vi "Dashboard Main.vi"() -> ()   [LabVIEW 2014]
uses:
  Program Files (x86)/National Instruments/LabVIEW 2014/examples/FRC/roboRIO/Vision/2015 Vision Example/Vision Support Code/Camera Types.ctl
  <vilib>/vision/Pattern Matching.llb/IMAQ Match Range Setting.ctl
  <vilib>/vision/Pattern Matching.llb/IMAQ Curve Parameters.ctl
  <vilib>/event_ctls.llb/eventvkey.ctl
  <vilib>/Rock Robotics/WPI/Dashboard/WPI_DashboardLogging Global.vi
  <vilib>/Utility/config.llb/Write Key (String).vi
  <vilib>/Utility/config.llb/Write Key (I32).vi
  <vilib>/Utility/config.llb/NI_LVConfig.lvlib
  <vilib>/vision/NI_Vision_Development_Module.lvlib
panel:
  out "Template 2":T1(plugin-control)
  in  "Camera Type":T2=enum."MS HD3000 square"
  out "ms to process":u32
  out "Particles":i32
  in  "TCP":refnum<k5>
  in  "Rec Mode":enum32{"Stop", "Record", "Playback"}(radio)
  in  "Vision":u16(ring) items=["Camera Off", "USB Camera SW", "USB Camera HW", "IP Camera"]
  out "Camera IP":string
  out "Image Message":string="Timeout in Camera Communications"
  in  "Dashboard Tab":T3(tab)
  in  "Camera Settings":T4={"Frame Rate"=30, "Compression"=30, "Size"=1} {"Frame Rate" scale=1.0..30.0; "Size" items=["640x480", "320x240", "160x120"]}
  out "MotorChart R":cluster{"Numeric":dbl, "Numeric":dbl}(graph)
  out "MotorChart L":T5(graph)
  out "MotorSliders R":cluster{"MotorSlide1":dbl, "MotorSlide2":dbl} {"MotorSlide2" scale=-1.0..1.0 scale format="%#_2e"; "MotorSlide1" scale=-1.0..1.0 scale format="%#_2e"}
  out "MotorSliders L":T6 {"MotorSlide4 2" scale=0.0..14.0 scale format="%#_2e"; "MotorSlide2" scale=-1.0..1.0 scale format="%#_2e"; "MotorSlide1" scale=-1.0..1.0 scale format="%#_2e"}
  out "Gyro":dbl(knob) scale=0.0..360.0
  out "JS1 Z":dbl(slide) scale=-1.0..1.0 scale format="%#_2e"
  out "JS1 Graph":cluster{"X":dbl, "Y":dbl}[](graph)
  out "JS1 Buttons":T7
  out "JS2 Z":dbl(slide) scale=-1.0..1.0 scale format="%#_2e"
  out "JS2 Graph":cluster{"X":dbl, "Y":dbl}[](graph)
  out "JS2 Buttons":T7
  out "Mode":T8(ring)=enum."Auto Disabled"
  in  "DB Camera Config":bool
  out "fps":dbl format="%#.1g"
  out "Mbps":dbl format="%#.1g"
  out "Mbps 2":bool
  in  "DB/String 9":string
  in  "DB/String 8":string
  in  "DB/String 7":string
  in  "DB/String 6":string
  in  "DB/String 5":string
  in  "DB/String 4":string
  in  "DB/String 3":string
  in  "DB/String 2":string
  in  "DB/String 1":string
  in  "DB/String 0":string
  in  "DB/Slider 0":dbl(slide) scale=0.0..5.0
  in  "DB/Slider 1":dbl(slide) scale=0.0..5.0
  in  "DB/Slider 2":dbl(slide) scale=0.0..5.0
  in  "DB/Slider 3":dbl(slide) scale=0.0..5.0
  out "DB/LED 3":bool
  out "DB/LED 2":bool
  out "DB/LED 1":bool
  out "DB/LED 0":bool
  in  "DB/Button 3":bool
  in  "DB/Button 2":bool
  in  "DB/Button 1":bool
  in  "DB/Button 0":bool caption="New Name"
  out "Scale":dbl
  out "Masked":T1(plugin-control)
  in  "Tote Color":T9={"Hue"={23.67058792990901, 48.923317529462665}, "Sat"={66.78571428571429, 255.0}, "Val"={48.571428571428584, 255.0}} {"Hue" scale=0.0..255.0 scale format="%#_3g"}
  out "Detected Totes":T10(array[cluster]) {"Normalized Rect"."Numeric 5" format="%#_2g"; "Normalized Rect"."Numeric 3" format="%#_2g"; "Normalized Rect"."Numeric 2" format="%#_2g"; "Normalized Rect"."Numeric" format="%#_2g"}
  out "Sorted Scores":T11(array[cluster]) {"Correlation" format="%#_3g"; "Scale %" format="%#_3g"; "Score" format="%#_3g"}
  in  "Annotate":bool=TRUE
  in  "Score Threshold":dbl=75.0
  out "RightSide":dbl
  out "LeftSide":dbl
  in  "Test Slider":dbl(slide) scale=0.0..100.0 scale format="%#_3g"
  in  "On/Off":bool caption="Solenoid"
  in  "Test Name":u16(ring) items=["Select the test to run...", "Example Test", "-------------------------------", "List of tests is built in robot code.", "Replace with your own automated tests."]
  in  "Test Tree":string(tree)
  in  "Motor":cluster{"Value":dbl, "Enable":bool} {"Value" scale=-1.0..1.0 scale format="%#_3g"}
  out "Progress":T12 {"Test Progress" scale=0.0..100.0}
  in  "Rev/Fwd":cluster{"Forward":bool, "Reverse":bool}
  in  "Test Ring":u16(ring) items=["Monochrome", "Color"]
  in  "Listbox":i32(listbox)
  out "Tree":string(tree)
  out "Camera Image":T1(plugin-control)
  out "Boolean":bool
  # "Left"
  # "Front"
  # "Right"
  # "Battery"
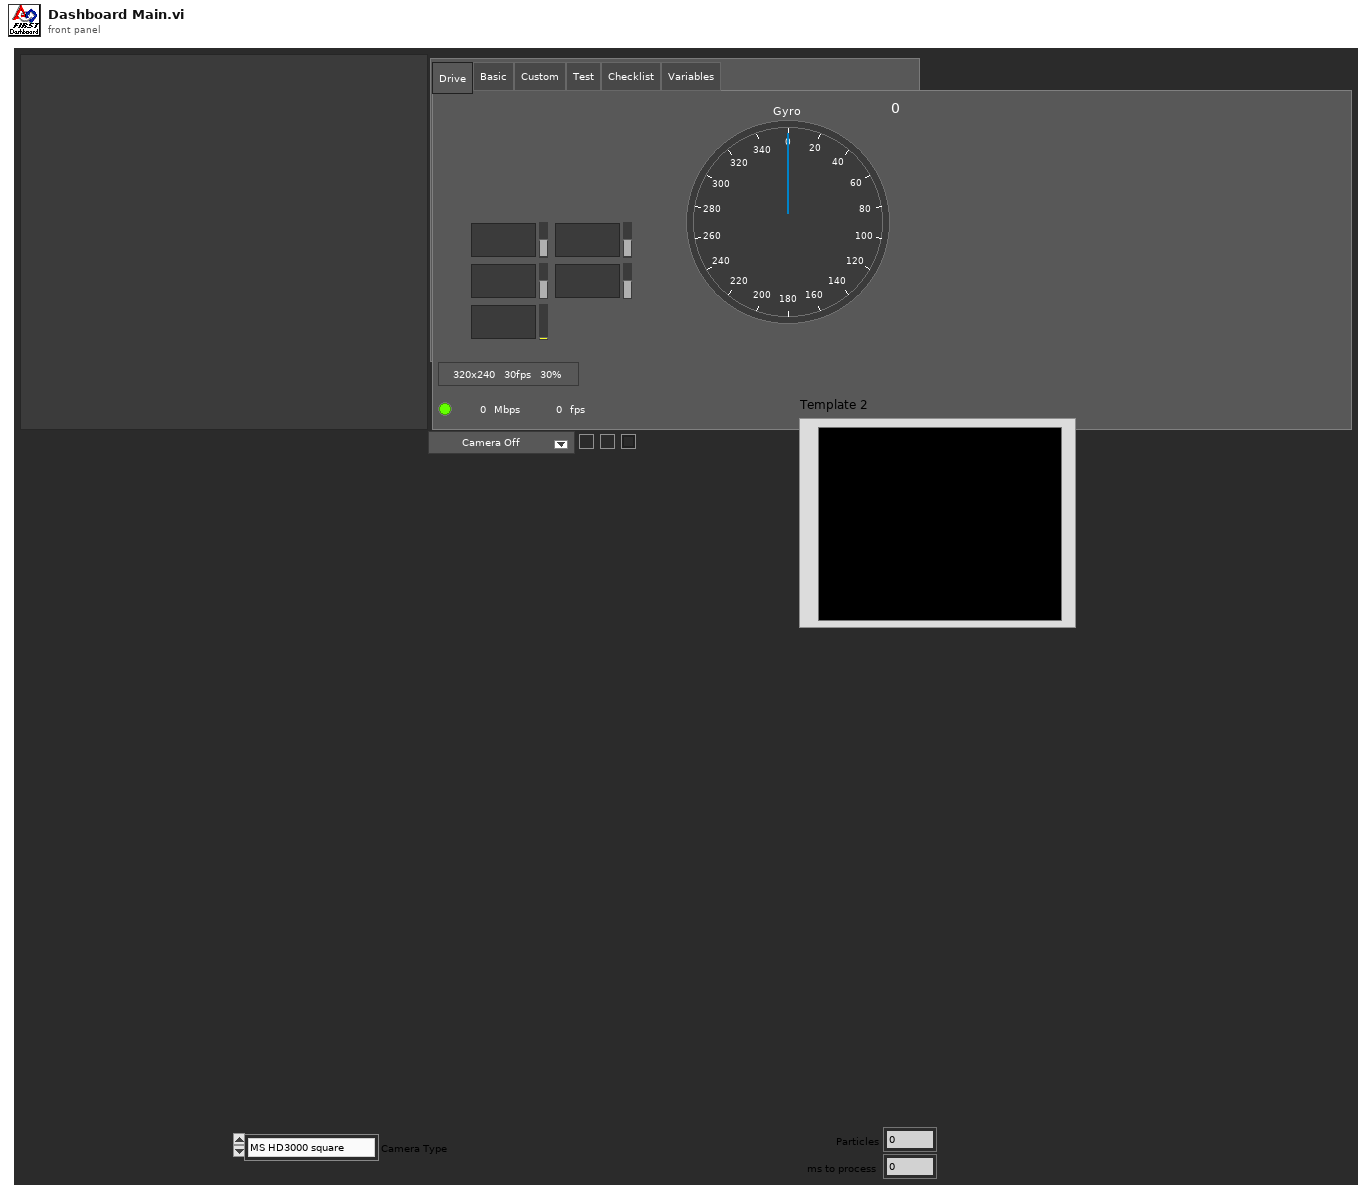
[diagram p1: front panel]
types:
  T1 = typedef "IMAQ Image.ctl" = refnum<image>
  T2 = typedef "Camera Types.ctl" = enum16{"206", "1011", "1013", "MS HD3000 square", "MS HD3000 640x480"}
  T3 = enum32{"Drive", "Basic", "Custom", "Test", "Checklist", "Variables"}
  T4 = cluster{"Frame Rate":i32, "Compression":i32, "Size":u16}
  T5 = cluster{"Numeric":dbl, "Numeric":dbl, "Battery V":dbl}
  T6 = cluster{"MotorSlide1":dbl, "MotorSlide2":dbl, "MotorSlide4 2":dbl}
  T7 = cluster{bool, bool, bool, bool, bool, bool, bool, bool, bool, bool, bool, bool}
  T8 = enum8{"Tele-Op Disabled", "Tele-Op Enabled", "Auto Disabled", "Auto Enabled", "Test Disabled", "Test Enabled", "Disconnected", "No Code", "E-Stop"}
  T9 = cluster{"Hue":cluster{dbl, dbl}, "Sat":cluster{dbl, dbl}, "Val":cluster{dbl, dbl}}
  T10 = cluster{"Distance (ft)":dbl, "Center":cluster{dbl, dbl}, "Normalized Rect":cluster{"Numeric":dbl, "Numeric 2":dbl, "Numeric 3":dbl, "Numeric 5":dbl}}[]
  T11 = cluster{"Rectangle":cluster{"Numeric":dbl, "Numeric 2":dbl, "Numeric 3":dbl, "Numeric 5":dbl}, "Scale %":dbl, "Score":dbl, "Correlation":dbl}[]
  T12 = cluster{"Test Progress":u8, "Test Progress Text":string}
  T13 = cluster{"Rotation":bool, "Scale":bool, "Occlusion":bool, "Reserved":bool, "Reserved":bool, "Reserved":bool}
  T14 = typedef "IMAQ Curve Parameters.ctl" = cluster{"Extraction Mode":u32, "Edge Threshold":i32, "Edge Filter Size":u32, "Min Length":i32, "Row Search Step Size":i32, "Col Search Step Size":i32, "Max Endpoint Gap":i32, "Closed":bool, "Subpixel":bool}
  T15 = typedef "IMAQ Match Range Setting.ctl" = cluster{"Match Constraints":u32, "Min":dbl, "Max":dbl}
  T16 = typedef "Image Type" = u32
  T17 = typedef "Particle Parameters" = i32
  T18 = cluster{"Error Strings":string, "Disable Counts":cluster{u16, u16}, "Rail Faults":cluster{u16, u16, u16}, "Robot IP":string, "DB Mode":u8, "Event Info":cluster{"Name":string, "Type":u8, "Number":u16, "Replay":u8}, "Camera Addr":string}
  T19 = cluster{"Storage":cluster{"Disk Free":u64, "RAM Block":u32, "RAM free":u32}, "CPU Utilization":cluster{"CPU % ISR":sgl, "CPU % Time Crit":sgl, "CPU % Timed Str":sgl, "CPU % High":sgl, "CPU % Above":sgl, "CPU % Normal":sgl, "CPU % Low":sgl}, "CAN":cluster{"% Bus Utilization":sgl, "Bus Off Cnt":u32, "TX_FIFO Full Cnt":u32, "Receive Error Cnt":u8, "Transmit Error Cnt":u8}, "HID":cluster{"HID Outputs":u32, "Rumble Low":u16, "Rumble High":u16}[]}
  T20 = cluster{"Status bits":cluster{"Test Mode":bool, "Autonomous":bool, "Enabled":bool, "Code Start":bool, "Brownout":bool, "Reserved 2":bool, "Reserved 3":bool, "E-Stop":bool}, "Code Trace":cluster{"Disabled":bool, "TeleOp":bool, "Auto":bool, "Test":bool}, "Controller Type":enum16{"unknown", "cRIO", "roboRio"}, "Code?":enum16{"unknown", "noCode", "code"}, "Battery V":dbl}
  T21 = cluster{"Control Bits":cluster{"TestMode":bool, "Autonomous":bool, "Enabled":bool, "FMS Present":bool, bool, bool, bool, "E-Stop":bool}, "Team Station ":u8, "Countdown":sgl, "Joystick Values":cluster{"Axes":dbl[], "Buttons":bool[], "POVs":i16[]}[]}
  T22 = cluster{"Axes":dbl[], "Buttons":bool[], "POVs":i16[]}[]
  T23 = cluster{"Axes":dbl[], "Buttons":bool[], "POVs":i16[]}
  T24 = cluster{"Buttons[0]":bool, "Buttons[1]":bool, "Buttons[2]":bool, "Buttons[3]":bool, "Buttons[4]":bool, "Buttons[5]":bool, "Buttons[6]":bool, "Buttons[7]":bool, "Buttons[8]":bool, "Buttons[9]":bool, "Buttons[10]":bool, "Buttons[11]":bool}
  T25 = cluster{"[0]":dbl, "[1]":dbl, "[2]":dbl, "[3]":dbl}
  T26 = cluster{"[0]":dbl, "[1]":dbl, "[2]":dbl, "[3]":dbl, "[4]":dbl}
  T27 = typedef "ROI Descriptor" = cluster{"Global Rectangle":i32[], "Contours":cluster{"ID":enum32{"External", "Internal"}, "Type":u32, "Coordinates":i32[]}[]}
  T28 = typedef "IMAQ GM Match Report.ctl" = cluster{"Position":cluster{"x":sgl, "y":sgl}, "Angle":sgl, "Scale":sgl, "Score":sgl, "Bounding Box":cluster{"x":sgl, "y":sgl}[], "Contrast Reversed":bool, "Occlusion %":sgl, "Template Target Curve Score":sgl, "Target Template Curve Score":sgl, "Correlation Score":sgl}
  T29 = cluster{cluster{"[0]":dbl, "[1]":dbl, "[2]":dbl, "[3]":dbl}, "Position":cluster{"x":sgl, "y":sgl}, "Bounding Box":cluster{"x":sgl, "y":sgl}[], "Scale":sgl, "Score":sgl, "Correlation Score":sgl}
  T30 = cluster{"Rectangle":cluster{"Numeric":dbl, "Numeric 2":dbl, "Numeric 3":dbl, "Numeric 5":dbl}, "Scale":dbl, "Score":dbl, "Correlation":dbl}[]
  T31 = cluster{"Found Totes[0]":cluster{"Distance (ft)":dbl, "Center":cluster{dbl, dbl}, "Normalized Rect":cluster{"Numeric":dbl, "Numeric 2":dbl, "Numeric 3":dbl, "Numeric 5":dbl}}, "Found Totes[1]":cluster{"Distance (ft)":dbl, "Center":cluster{dbl, dbl}, "Normalized Rect":cluster{"Numeric":dbl, "Numeric 2":dbl, "Numeric 3":dbl, "Numeric 5":dbl}}, "Found Totes[2]":cluster{"Distance (ft)":dbl, "Center":cluster{dbl, dbl}, "Normalized Rect":cluster{"Numeric":dbl, "Numeric 2":dbl, "Numeric 3":dbl, "Numeric 5":dbl}}, "Found Totes[3]":cluster{"Distance (ft)":dbl, "Center":cluster{dbl, dbl}, "Normalized Rect":cluster{"Numeric":dbl, "Numeric 2":dbl, "Numeric 3":dbl, "Numeric 5":dbl}}, "Found Totes[4]":cluster{"Distance (ft)":dbl, "Center":cluster{dbl, dbl}, "Normalized Rect":cluster{"Numeric":dbl, "Numeric 2":dbl, "Numeric 3":dbl, "Numeric 5":dbl}}, "Found Totes[5]":cluster{"Distance (ft)":dbl, "Center":cluster{dbl, dbl}, "Normalized Rect":cluster{"Numeric":dbl, "Numeric 2":dbl, "Numeric 3":dbl, "Numeric 5":dbl}}, "Found Totes[6]":cluster{"Distance (ft)":dbl, "Center":cluster{dbl, dbl}, "Normalized Rect":cluster{"Numeric":dbl, "Numeric 2":dbl, "Numeric 3":dbl, "Numeric 5":dbl}}, "Found Totes[7]":cluster{"Distance (ft)":dbl, "Center":cluster{dbl, dbl}, "Normalized Rect":cluster{"Numeric":dbl, "Numeric 2":dbl, "Numeric 3":dbl, "Numeric 5":dbl}}, "Found Totes[8]":cluster{"Distance (ft)":dbl, "Center":cluster{dbl, dbl}, "Normalized Rect":cluster{"Numeric":dbl, "Numeric 2":dbl, "Numeric 3":dbl, "Numeric 5":dbl}}}
  T32 = cluster{"Distance (ft)":dbl, "Center":cluster{dbl, dbl}, "Normalized Rect":cluster{"Numeric":dbl, "Numeric 2":dbl, "Numeric 3":dbl, "Numeric 5":dbl}}
  T33 = cluster{"Sorted Scores[0]":cluster{"Rectangle":cluster{"Numeric":dbl, "Numeric 2":dbl, "Numeric 3":dbl, "Numeric 5":dbl}, "Scale":dbl, "Score":dbl, "Correlation":dbl}, "Sorted Scores[1]":cluster{"Rectangle":cluster{"Numeric":dbl, "Numeric 2":dbl, "Numeric 3":dbl, "Numeric 5":dbl}, "Scale":dbl, "Score":dbl, "Correlation":dbl}, "Sorted Scores[2]":cluster{"Rectangle":cluster{"Numeric":dbl, "Numeric 2":dbl, "Numeric 3":dbl, "Numeric 5":dbl}, "Scale":dbl, "Score":dbl, "Correlation":dbl}, "Sorted Scores[3]":cluster{"Rectangle":cluster{"Numeric":dbl, "Numeric 2":dbl, "Numeric 3":dbl, "Numeric 5":dbl}, "Scale":dbl, "Score":dbl, "Correlation":dbl}, "Sorted Scores[4]":cluster{"Rectangle":cluster{"Numeric":dbl, "Numeric 2":dbl, "Numeric 3":dbl, "Numeric 5":dbl}, "Scale":dbl, "Score":dbl, "Correlation":dbl}, "Sorted Scores[5]":cluster{"Rectangle":cluster{"Numeric":dbl, "Numeric 2":dbl, "Numeric 3":dbl, "Numeric 5":dbl}, "Scale":dbl, "Score":dbl, "Correlation":dbl}, "Sorted Scores[6]":cluster{"Rectangle":cluster{"Numeric":dbl, "Numeric 2":dbl, "Numeric 3":dbl, "Numeric 5":dbl}, "Scale":dbl, "Score":dbl, "Correlation":dbl}, "Sorted Scores[7]":cluster{"Rectangle":cluster{"Numeric":dbl, "Numeric 2":dbl, "Numeric 3":dbl, "Numeric 5":dbl}, "Scale":dbl, "Score":dbl, "Correlation":dbl}, "Sorted Scores[8]":cluster{"Rectangle":cluster{"Numeric":dbl, "Numeric 2":dbl, "Numeric 3":dbl, "Numeric 5":dbl}, "Scale":dbl, "Score":dbl, "Correlation":dbl}}
  T34 = cluster{"Rectangle":cluster{"Numeric":dbl, "Numeric 2":dbl, "Numeric 3":dbl, "Numeric 5":dbl}, "Scale":dbl, "Score":dbl, "Correlation":dbl}
  T35 = cluster{"Numeric":dbl, "Numeric 2":dbl, "Numeric 3":dbl, "Numeric 5":dbl}
  T36 = typedef "NI_LVConfig.lvlib/Config Data RefNum.ctl" = refnum<k1>
  T37 = cluster{"Operation":enum16{"Update", "Clear"}, "Color Box":u32}[]
  T38 = typedef "eventvkey.ctl" = enum16{"ASCII", "Enter", "Return", "Shift", "Ctrl", "Alt", "Cmd", "Opt", "Caps", "NumLock", "Clear", "Break", "Up", "Down", "Left", "Right", "Insert", "Delete", "Home", "End", "PageUp", "PageDown", "Escape", "Help", "Pause", "ScrollLock", "F1", "F2", "F3", "F4", "F5", "F6", "F7", "F8", "F9", "F10", "F11", "F12", "F13", "F14", "F15", "F16", "F17", "F18", "F19", "F20", "F21", "F22", "F23", "F24", "Play", "VolumeUp", "VolumeDown", "Mute", "Two Byte Char"}
  T39 = cluster{"Image Size":bool, "Image Type":bool, "Pixel Value":bool, "ROI Information":bool, "Zoom Factor":bool}
  T40 = enum8{"Enabled", "Disabled", "Disabled and Grayed Out"}
  T41 = cluster{"Operation":enum16{"Update", "Clear"}, "Color Box":u32}
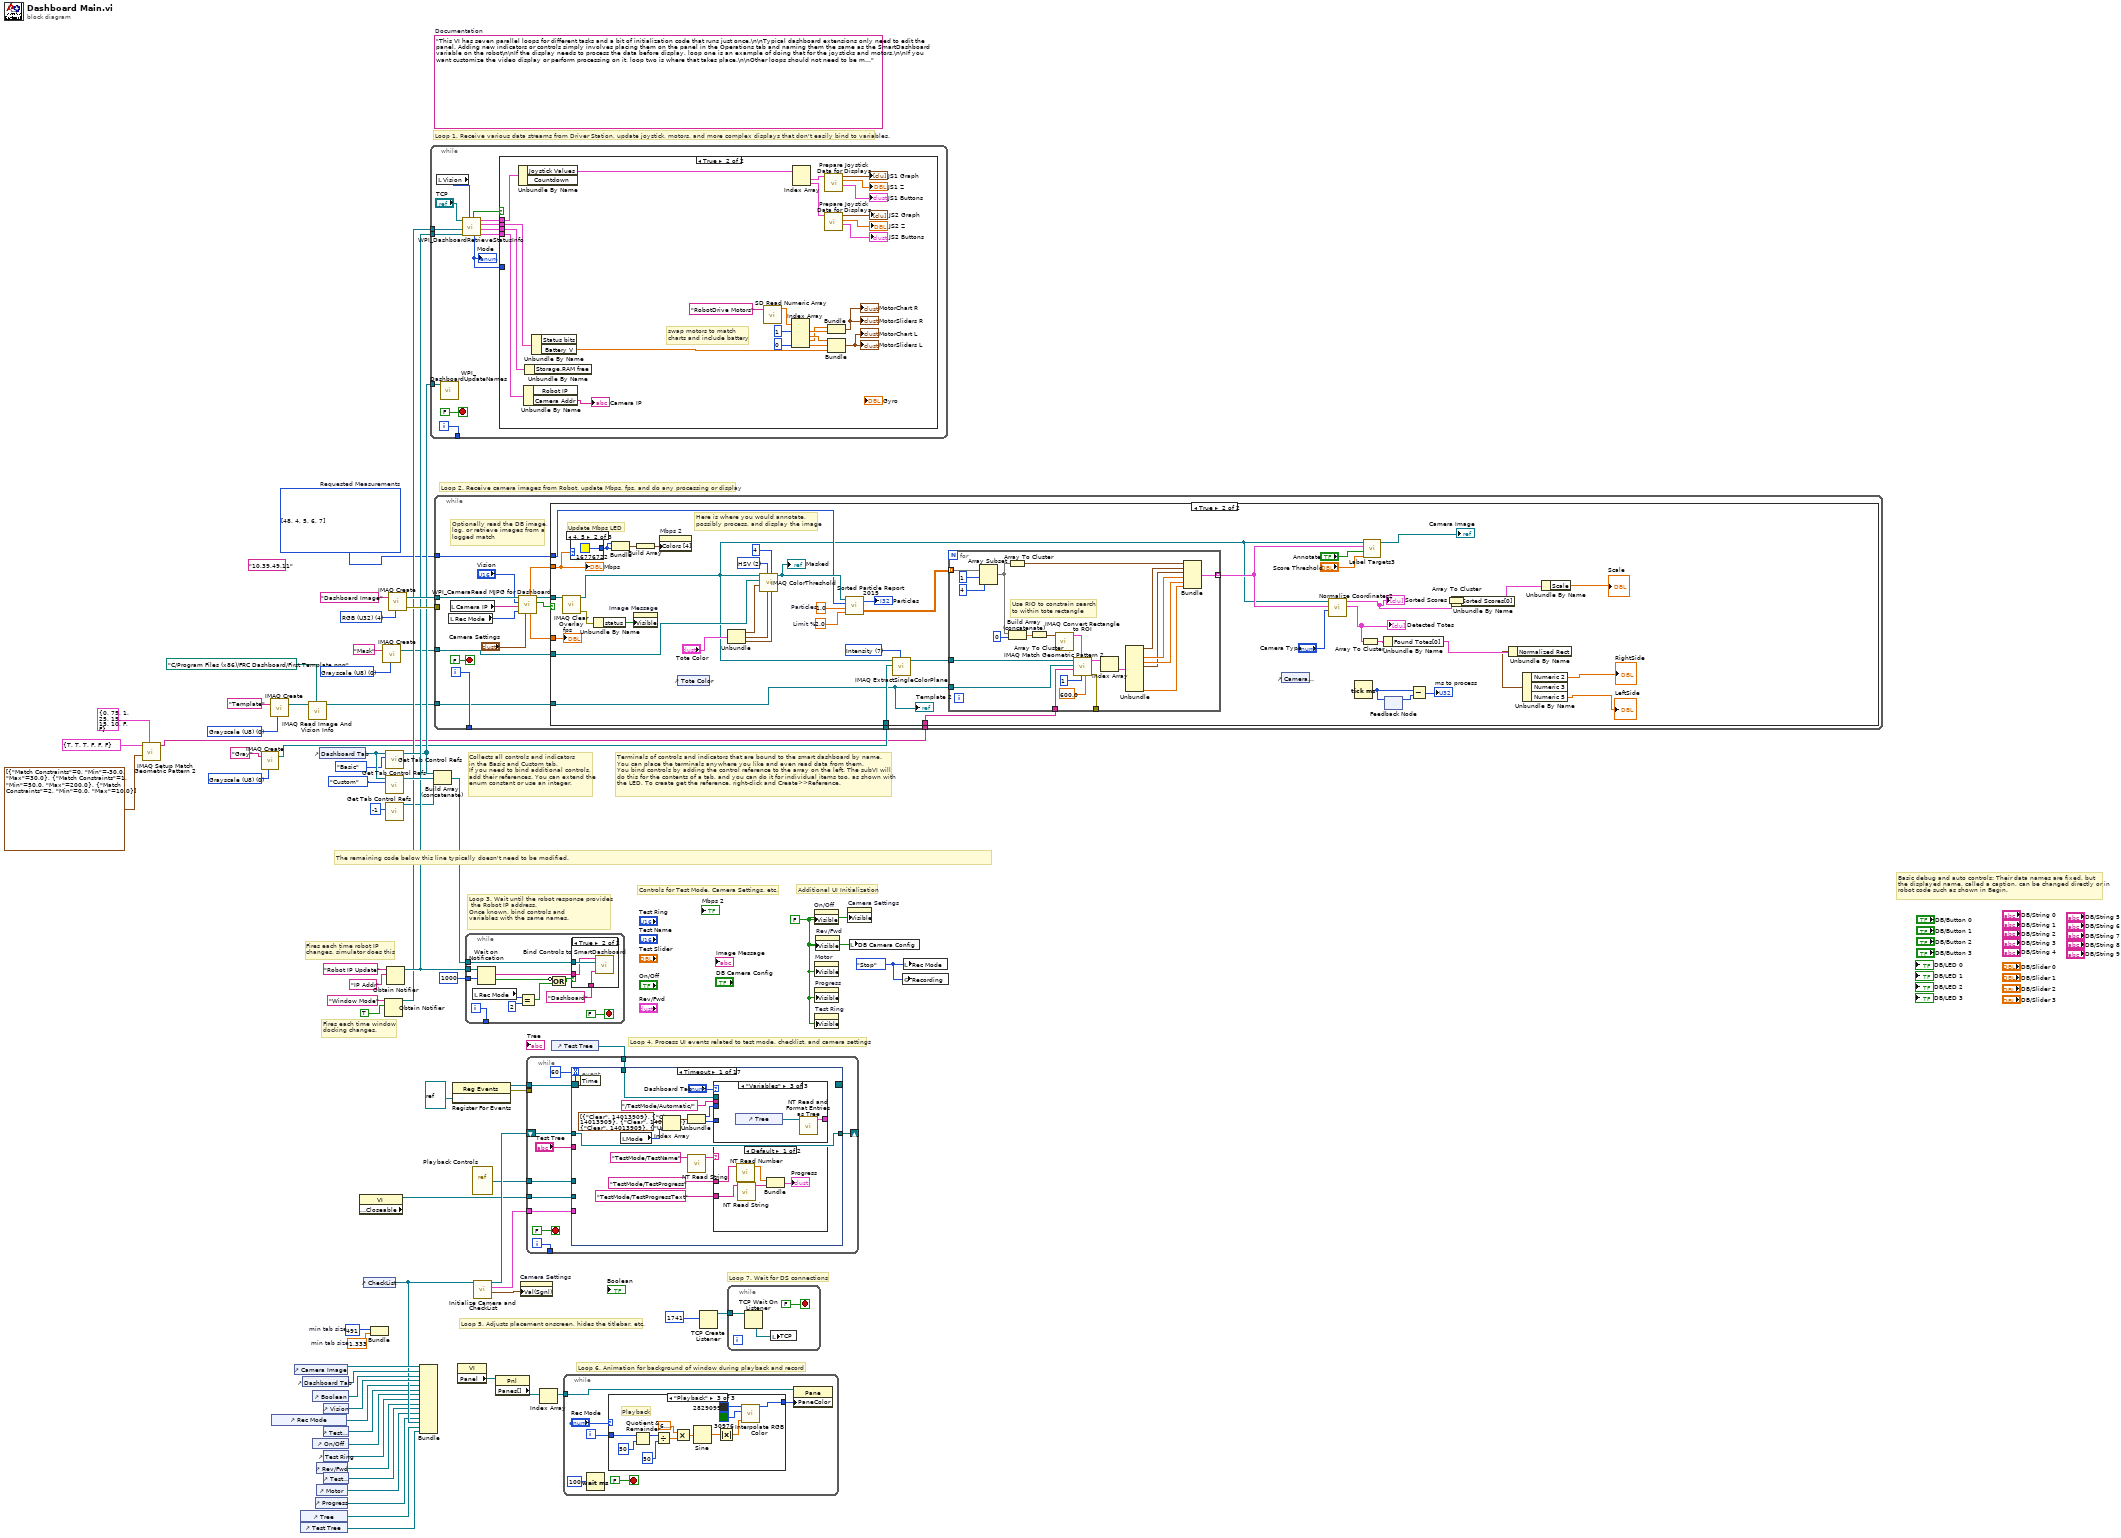
[diagram p0: block diagram]
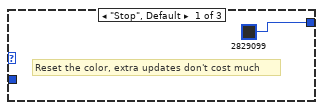
[diagram p3: hidden frame]
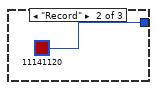
[diagram p4: hidden frame]
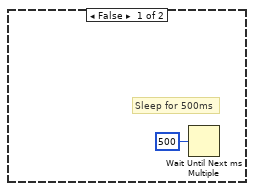
[diagram p6: hidden frame]
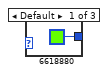
[diagram p7: hidden frame]
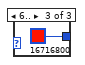
[diagram p8: hidden frame]
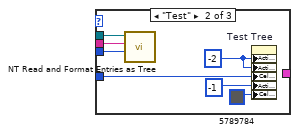
[diagram p10: hidden frame]
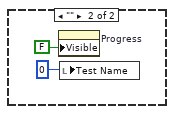
[diagram p11: hidden frame]
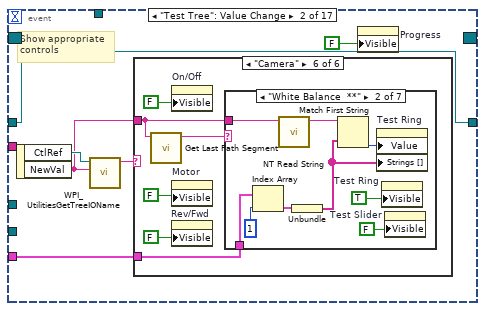
[diagram p12: hidden frame]
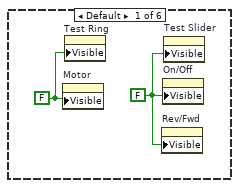
[diagram p13: hidden frame]
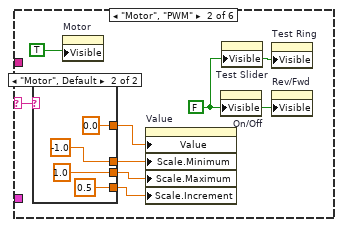
[diagram p14: hidden frame]
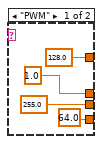
[diagram p15: hidden frame]
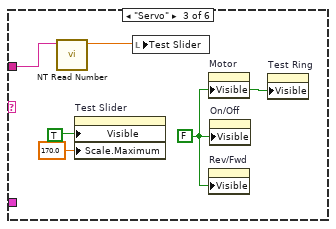
[diagram p16: hidden frame]
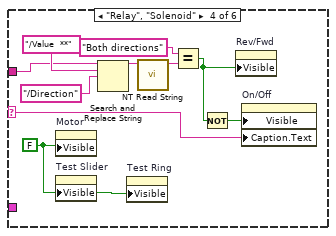
[diagram p17: hidden frame]
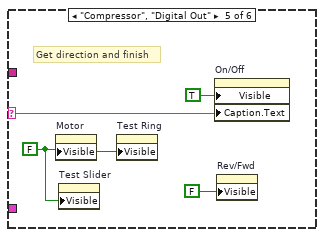
[diagram p18: hidden frame]
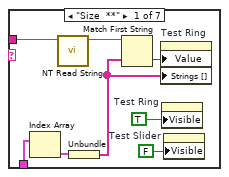
[diagram p19: hidden frame]
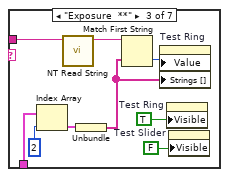
[diagram p20: hidden frame]
diagram:
  (unwired) "10.39.49.11" ("Camera IP")
  w10 = T16 0 items=["Grayscale (U8)", "Grayscale (I16)", "Grayscale (SGL)", "Complex (CSG)", "RGB (U32)", "HSL (U32)", "RGB (U64)", "Grayscale (U16)"] ("Image Type")
  w14 = T16 0 items=["Grayscale (U8)", "Grayscale (I16)", "Grayscale (SGL)", "Complex (CSG)", "RGB (U32)", "HSL (U32)", "RGB (U64)", "Grayscale (U16)"] ("Image Type")
  w15 = T17[] [48, 4, 5, 6, 7] items=["Center of Mass X", "Center of Mass Y", "First Pixel X", "First Pixel Y", "Bounding Rect Left", "Bounding Rect Top", "Bounding Rect Right", "Bounding Rect Bottom", "Max Feret Diameter Start X", "Max Feret Diameter Start Y", "Max Feret Diameter End X", "Max Feret Diameter End Y", "Max Horiz. Segment Length Left", "Max Horiz. Segment Length Right", "Max Horiz. Segment Length Row", "-", "Bounding Rect Width", "Bounding Rect Height", "Bounding Rect Diagonal", "Perimeter", "Convex Hull Perimeter", "Holes' Perimeter", "Max Feret Diameter", "Equivalent Ellipse Major Axis", "Equivalent Ellipse Minor Axis", "Equivalent Ellipse Minor Axis (Feret)", "Equivalent Rect Long Side", "Equivalent Rect Short Side", "Equivalent Rect Diagonal", "Equivalent Rect Short Side (Feret)", "Average Horiz. Segment Length", "Average Vert. Segment Length", "Hydraulic Radius", "Waddel Disk Diameter", "-", "Area", "Holes' Area", "Particle & Holes' Area", "Convex Hull Area", "Image Area", "-", "Number of Holes", "Number of Horiz. Segments", "Number of Vert. Segments", "-", "Orientation", "Max Feret Diameter Orientation", "-", "% Area/Image Area", "% Area/(Particle & Holes' Area)", "Ratio of Equivalent Ellipse Axes", "Ratio of Equivalent Rect Sides", "-", "Elongation Factor", "Compactness Factor", "Heywood Circularity Factor", "Type Factor", "-", "Sum X", "Sum Y", "Sum XX", "Sum XY", "Sum YY", "Sum XXX", "Sum XXY", "Sum XYY", "Sum YYY", "-", "Moment of Inertia XX", "Moment of Inertia XY", "Moment of Inertia YY", "Moment of Inertia XXX", "Moment of Inertia XXY", "Moment of Inertia XYY", "Moment of Inertia YYY", "Norm. Moment of Inertia XX", "Norm. Moment of Inertia XY", "Norm. Moment of Inertia YY", "Norm. Moment of Inertia XXX", "Norm. Moment of Inertia XXY", "Norm. Moment of Inertia XYY", "Norm. Moment of Inertia YYY", "Hu Moment 1", "Hu Moment 2", "Hu Moment 3", "Hu Moment 4", "Hu Moment 5", "Hu Moment 6", "Hu Moment 7"]  # Requested Measurements
  w18 = T16 0 items=["Grayscale (U8)", "Grayscale (I16)", "Grayscale (SGL)", "Complex (CSG)", "RGB (U32)", "HSL (U32)", "RGB (U64)", "Grayscale (U16)"] ("Image Type")
  w40 = 491  # min tab size
  w39 = 1.333  # min tab size
  w48 = enum32{"Stop", "Record", "Playback"}."Stop" ("Rec Mode")
  w24 = FALSE ("Visible")
  (unwired) "This VI has seven parallel loops for different tasks and a bit of initialization code that runs just once.\n\nTypical dashboard extensions only need to edit the panel. Adding new indicators or controls simply involves placing them on the panel in the Operations tab and naming them the same as the SmartDashboard variable on the robot\n\nIf the display needs to process the data before display, loop one is an example of doing that for the joysticks and motors.\n\nIf you want customize the video display or perform processing on it, loop two is where that takes place.\n\nOther loops should not need to be modified. They are pretty standard, and document the task they perform."  # Documentation
  w68 = T16 4 items=["Grayscale (U8)", "Grayscale (I16)", "Grayscale (SGL)", "Complex (CSG)", "RGB (U32)", "HSL (U32)", "RGB (U64)"] ("Image Type")
  # "Loop 7. Wait for DS connections"
  # "Basic debug and auto controls: Their data names are fixed, but\nthe displayed name, called a caption, can be changed directly or in\nrobot code such as shown in Begin."
  # "Controls for Test Mode, Camera Settings, etc."
  # "Additional UI Initialization"
  # "Loop 6. Animation for background of window during playback and record"
  # "Fires each time robot IP\nchanges, simulator does this"
  # "Fires each time window\ndocking changes."
  # "Collects all controls and indicators\nin the Basic and Custom tab.\nIf you need to bind additional controls,\nadd their references. You can extend the\nenum constant or use an integer."
  # "The remaining code below this line typically doesn't need to be modified."
  # "Loop 4. Process UI events related to test mode, checklist, and camera settings"
  # "Terminals of controls and indicators that are bound to the smart dashboard by name.\nYou can place the terminals anywhere you like and even read data from them.\nYou bind controls by adding the control reference to the array on the left. The subVI will\ndo this for the contents of a tab, and you can do it for individual items too, as shown with\nthe LED. To create get the reference, right-click and Create>>Reference."
  # "Loop 3. Wait until the robot response provides\n the Robot IP address.\nOnce known, bind controls and\nvariables with the same names."
  # "Loop 5. Adjusts placement onscreen, hides the titlebar, etc."
  # "Loop 1. Receive various data streams from Driver Station, update joystick, motors, and more complex displays that don't easily bind to variables."
  # "Loop 2. Receive camera images from Robot, update Mbps, fps, and do any processing or display"
  n1 = call "IMAQ Setup Match Geometric Pattern 2"("Curve Parameters"=T14 {"Extraction Mode"=0, "Edge Threshold"=75, "Edge Filter Size"=1, "Min Length"=25, "Row Search Step Size"=15, "Col Search Step Size"=15, "Max Endpoint Gap"=10, "Closed"=FALSE, "Subpixel"=FALSE}, "Range Settings"=T15[] [{"Match Constraints"=0, "Min"=-30.0, "Max"=30.0}, {"Match Constraints"=1, "Min"=50.0, "Max"=200.0}, {"Match Constraints"=2, "Min"=0.0, "Max"=10.0}], "Match Mode"=T13 {"Rotation"=TRUE, "Scale"=TRUE, "Occlusion"=TRUE, "Reserved"=FALSE, "Reserved"=FALSE, "Reserved"=FALSE}) -> ("Match Geometric Pattern 2 Setup Data"=w4:string)  [unwired: 7 in, 1 out]
  n2 = call "IMAQ Create"("Image Name"="Gray", "Image Type"=w10) -> ("New Image"=w8:T1)  [unwired: 2 in, 2 out]
  n3 = call "IMAQ Create"("Image Name"="Template", "Image Type"=w14) -> ("New Image"=w12:T1)  [unwired: 2 in, 2 out]
  n4 = control-ref of="Rec Mode"() -> (w30:refnum<vi>)
  n5 = control-ref of="Camera Image"() -> (w43:refnum<vi>)
  n6 = control-ref of="Tree"() -> (w34:refnum<vi>)
  n7 = control-ref of="Test Tree"() -> (w33:refnum<vi>)
  n8 = control-ref of="Dashboard Tab"() -> (w42:refnum<vi>)
  n9 = call "IMAQ Read Image And Vision Info"("File Path"=path "C:/Program Files (x86)/FRC Dashboard/First Template.png", "Image"=w12) -> ("Image Out"=w11:T1)  [unwired: 2 in, 7 out]
  n10 = control-ref of="Boolean"() -> (w38:refnum<vi>)
  n11 = control-ref of="On/Off"() -> (w28:refnum<vi>)
  n12 = control-ref of="Progress"() -> (w25:refnum<vi>)
  n13 = control-ref of="Rev/Fwd"() -> (w26:refnum<vi>)
  n14 = control-ref of="Motor"() -> (w31:refnum<vi>)
  n15 = control-ref of="Dashboard Tab"() -> (w46:refnum<vi>)
  n16 = control-ref of="Test Slider"() -> (w29:refnum<vi>)
  n17 = control-ref of="Vision"() -> (w41:refnum<vi>)
  n18 = control-ref of="Test Ring"() -> (w27:refnum<vi>)
  n19 = control-ref of="Test Name"() -> (w32:refnum<vi>)
  n20 = property class="VI" props=["Front Panel.Closeable"]() -> (reference out=w47:refnum<vi>)  [unwired: 2 in, 2 out]
  n21 = control-ref of="CheckList"() -> (w35:refnum<vi>)
  n22 = Bundle("min tab size"=w40, "min tab size"=w39) -> ()  [unwired: 1 in, 1 out]
  n23 = call "IMAQ Create"("Image Name"="Mask", "Image Type"=w18) -> ("New Image"=w16:T1)  [unwired: 2 in, 2 out]
  n24 = Obtain Notifier(name (unnamed)="Window Mode", notification data type=TRUE) -> (notifier out=w21:refnum<notifier>)  [unwired: 2 in, 2 out]
  n25 = call <vilib>:"Get Tab Control Refs.vi"("Page Index"=T3."Basic" ("Dashboard Tab"), "TabControl in"=w46) -> ("ControlsOnPage"=w22:refnum<vi>[])  [unwired: 9 in]
  n26 = call <vilib>:"Get Tab Control Refs.vi"("Page Index"=T3."Custom" ("Dashboard Tab"), "TabControl in"=w46) -> ("ControlsOnPage"=w45:refnum<vi>[])  [unwired: 9 in]
  n27 = call <vilib>:"Get Tab Control Refs.vi"("Page Index"=-1) -> ("ControlsOnPage"=w2:refnum<vi>[])  [unwired: 10 in]
  n28 = Obtain Notifier(name (unnamed)="Robot IP Update", notification data type="IP Addr" ("name (unnamed)")) -> (notifier out=w23:refnum<notifier>)  [unwired: 2 in, 2 out]
  n29 = call "IMAQ Create"("Image Name"="Dashboard Image", "Image Type"=w68) -> ("New Image"=w66:T1, "error out"=w65:errorcluster)  [unwired: 2 in, 1 out]
  n30 = Bundle("Camera Image"=w43, "Dashboard Tab"=w42, "Boolean"=w38, "Vision"=w41, "Rec Mode"=w30, "Test Slider"=w29, "On/Off"=w28, "Test Ring"=w27, "Rev/Fwd"=w26, "Test Name"=w32, "Motor"=w31, "Progress"=w25, "CheckList"=w35, "Tree"=w34, "Test Tree"=w33) -> ()  [unwired: 1 in, 1 out]
  n31 = while {
    tunnel: [w80] -> _
    tunnel: w23 -> [w74]
    tunnel: w22 -> [w73]
    tunnel: w21 -> [w69]
    i -> [w80]
    stop <- FALSE stop-if-true
    n32 = local read "Vision"() -> (w71:u16)
    n33 = call <vilib>:"WPI_DashboardUpdateNames.vi"("Controls on Tab"=w73) -> ()  [unwired: 11 in]
    n34 = call <vilib>:"WPI_DashboardRetrieveStatusInfo.vi"("Vision"=w71, "Binding Refnum"=w74, "Window Mode Notifier"=w69, "TCP Cnx"="TCP") -> ("Power and Errors"=w75:T18, "Robot Metrics"=w78:T19, "Status Info"=w79:T20, "Control Info"=w76:T21, "Robot Mode"=w72:T8, "Process?"=w77:bool)  [unwired: 2 in]
    "Mode" <- w72
    n35 = case shown="True" w77 {
      tunnel: w79 -> [_ w106]
      tunnel: w78 -> [_ w105]
      tunnel: w76 -> [_ w104]
      tunnel: w75 -> [_ w103]
      tunnel: w72 -> [_ _]
      frame False {
      }
      frame True {
        # "swap motors to match\ncharts and include battery"
        n36 = Unbundle By Name(w104) -> ("Joystick Values"=w91:T22)  [unwired: 1 out]
        n37 = Unbundle By Name(w103) -> ("Camera Addr"=→"Camera IP":string)  [unwired: 1 out]
        n38 = Unbundle By Name(w105) -> ()  [unwired: 1 out]
        n39 = Unbundle By Name(w106) -> ("Battery V"=w92:dbl)  [unwired: 1 out]
        n40 = call <vilib>:"SD Read Numeric Array.vi"("Name"="RobotDrive Motors") -> ("Numeric Array"=w94:dbl[])  [unwired: 8 in, 2 out]
        n41 = Index Array(array=w94, index #1=1, index #4=0) -> (element #1=w98:dbl, element #2=w99:dbl, element #3=w97:dbl, element #4=w102:dbl)  [unwired: 2 in]
        n42 = Index Array(array=w91) -> (element #1=w90:T23, element #2=w85:T23)  [unwired: 2 in]
        n43 = call "Prepare Joystick Data for Displays.vi"("Joystick Values"=w85) -> ("Buttons"=→"JS2 Buttons":T24, "Z Axis"=→"JS2 Z":dbl, "Cartesian Data"=→"JS2 Graph":cluster{"X axis":dbl, "X axis":dbl}[])  [unwired: 8 in]
        n44 = call "Prepare Joystick Data for Displays.vi"("Joystick Values"=w90) -> ("Buttons"=→"JS1 Buttons":T24, "Z Axis"=→"JS1 Z":dbl, "Cartesian Data"=→"JS1 Graph":cluster{"X axis":dbl, "X axis":dbl}[])  [unwired: 8 in]
        n45 = Bundle("Numeric"=w97, "Numeric"=w98) -> (→"MotorChart R" →"MotorSliders R":cluster{"Numeric":dbl, "Numeric":dbl})  [unwired: 1 in]
        n46 = Bundle("Numeric"=w99, "Numeric"=w102, "Battery V"=w92) -> (→"MotorChart L" →"MotorSliders L":T5)  [unwired: 1 in]
      }
    }
  }
  n47 = Build Array (concatenate)(w22, w45, w2) -> (w44:refnum<vi>[])
  n48 = while {
    tunnel: w66 -> [w120]
    tunnel: w65 -> [_]
    tunnel: [w121] -> _
    tunnel: w16 -> [w112]
    tunnel: w15 -> [w111]
    tunnel: w11 -> [w110]
    tunnel: w8 -> [w109]
    tunnel: w4 -> [w108]
    i -> [w121]
    stop <- FALSE stop-if-true
    # "Optionally read the DB image,\nlog, or retrieve images from a\nlogged match"
    n49 = local read "Rec Mode"() -> (w114:enum32{"Stop", "Record", "Playback"})
    n50 = local read "Camera IP"() -> (w107:string)
    n51 = call <vilib>:"WPI_CameraRead MJPG for Dashboard.vi"("Camera Settings"="Camera Settings", "Rec Mode"=w114, "Camera IP"=w107, "Camera Mode"="Vision", "Refnum in"=w120) -> ("Active"=w118:bool, "Refnum out"=w119:T1, "FPS"=w117:dbl, "Bandwidth (Mbps)"=w116:dbl)  [unwired: 3 in]
    n52 = case shown="True" w118 {
      tunnel: w119 -> [_ w163]
      tunnel: w116 -> [_ w162]
      tunnel: w117 -> [_ w161]
      tunnel: w112 -> [_ w139]
      tunnel: w111 -> [_ w138]
      tunnel: w110 -> [_ w134]
      tunnel: w109 -> [_ w136]
      tunnel: w108 -> [_ w135]
      frame False {
        # "Sleep for 500ms"
        n53 = Wait Until Next ms Multiple(millisecond multiple=u32 500) -> ()  [unwired: 1 out]
      }
      frame True {
        w149 = 7 items=["Red", "Green", "Blue", "Hue", "Saturation", "Luminance", "Value", "Intensity"] ("Color Plane")
        w154 = 2.0  # Limit %
        w156 = 1.0  # Particles
        w160 = u16 2 items=["RGB", "HSL", "HSV", "HSI"] ("Color Mode")
        # "Here is where you would annotate,\npossibly process, and display the image"
        # "Update Mbps LED"
        n54 = call "IMAQ Clear Overlay"("Image"=w163) -> ("error out"=w167:errorcluster, "Image Out"=w137:T1)  [unwired: 2 in, 7 out]
        n55 = case shown="4, 5" w162 {
          tunnel: [u32 6618880 ("Color Box") u32 16776722 ("Color Box") u32 16716800 ("Color Box")] -> w164
          frame Default {
          }
          frame 4, 5 {
          }
          frame 6.. {
          }
        }
        n56 = Unbundle By Name(w167) -> ("status"=w168:bool)
        n57 = Bundle("Color Box"=w164, "Color Box"=w164) -> (w166:cluster{"Color Box":u32, "Color Box":u32})  [unwired: 1 out]
        n58 = property on="Image Message" class="Str"("Visible"=w168) -> ()  [unwired: 2 in, 2 out]
        n59 = Build Array(w166) -> (w165:cluster{"Color Box":u32, "Color Box":u32}[])
        n60 = property on="Mbps 2" class="Bool (strict)"("Colors [4]"=w165) -> ()  [unwired: 2 in, 2 out]
        n61 = control-ref of="Tote Color"() -> ()  [unwired: 1 out]
        n62 = Unbundle("Tote Color") -> ("Hue"=w159:cluster{dbl, dbl}, "Sat"=w158:cluster{dbl, dbl}, "Val"=w157:cluster{dbl, dbl})
        n63 = call "IMAQ ColorThreshold"("Blue or Luma or Val or Inten Range"=w157, "Replace Value"=4, "Green or Sat Range"=w158, "Color Mode"=w160, "Red or Hue Range"=w159, "Image Dst"=w139, "Image Src"=w137) -> ("Image Dst Out"=w148:T1)  [unwired: 3 in, 1 out]
        "Masked" <- w148
        n64 = call "Sorted Particle Report 2015.vi"("Min Area Size %"=w154, "Particle Count Limit"=w156, "Pixel Measurements"=w138, "Image in"=w148) -> ("Sorted Data"=w146:dbl[][], "Particles"=→"Particles":i32)
        n65 = call "IMAQ ExtractSingleColorPlane"("Color Plane"=w149, "Image Dst"=w136, "Image Src"=w137) -> ("Image Dst Out"=w147:T1)  [unwired: 7 in, 1 out]
        n66 = for {
          tunnel: w146 -> [w189] mode=indexing
          tunnel: [w188] -> w143 mode=indexing
          tunnel: w147 -> [w179]
          tunnel: w135 -> [w181]
          tunnel: w134 -> [w171]
          tunnel: [w170] -> _
          # "Use RIO to constrain search\nto within tote rectangle"
          n67 = Array Subset(array=w189, index=1, length=4) -> (w182:dbl[])
          n68 = Array To Cluster(array=w182) -> (cluster=w183:T25)
          n69 = Build Array (concatenate)(w182, 0 ("length")) -> (w186:dbl[])
          n70 = Array To Cluster(array=w186) -> (cluster=w185:T26)
          n71 = call "IMAQ Convert Rectangle to ROI"("Rectangle"=w185) -> ("ROI Descriptor"=w184:T27)  [unwired: 8 in, 1 out]
          n72 = call "IMAQ Match Geometric Pattern 2"("Minimum Match Score"=sgl 600.0, "Number of Matches Requested"=1 ("Minimum Match Score"), "ROI Descriptor"=w184, "Match Geometric Pattern 2 Setup Data"=w181, "Template Image"=w171, "Image"=w179) -> ("error out"=w170:errorcluster, "Matches (pixel)"=w177:T28[])  [unwired: 2 in, 2 out]
          n73 = Index Array(array=w177) -> (element=w176:T28)  [unwired: 1 in]
          n74 = Unbundle(w176) -> ("Position"=w175:cluster{"x":sgl, "y":sgl}, "Scale"=w174:sgl, "Score"=w173:sgl, "Bounding Box"=w169:cluster{"x":sgl, "y":sgl}[], "Correlation Score"=w172:sgl)  [unwired: 5 out]
          n75 = Bundle(w183, "Position"=w175, "Bounding Box"=w169, "Scale"=w174, "Score"=w173, "Correlation Score"=w172) -> (w188:T29)  [unwired: 1 in]
        }
        n76 = control-ref of="Camera Type"() -> ()  [unwired: 1 out]
        n77 = call "Normalize Coordinates2.vi"("Camera Type"="Camera Type", "Targets"=w143, "Image in"=w137) -> ("Found Totes"=w130:T10, "Sorted Scores"=w133:T30)  [unwired: 7 in]
        "Sorted Scores" <- w133
        "Detected Totes" <- w130
        n78 = Tick Count (ms)() -> (millisecond timer value=w152:u32)
        n79 = Array To Cluster(array=w130) -> (cluster=w129:T31)
        n80 = call "Label Targets3.vi"("Score Threshold"="Score Threshold", "Annotate"="Annotate", "Targets"=w143, "Image in"=w137) -> ("Image out"=→"Camera Image":T1)  [unwired: 7 in]
        n81 = Unbundle By Name(w129) -> ("Found Totes[0]"=w128:T32)
        n82 = feedback #1() -> (w153:u32)  [unwired: 1 in]
        n83 = feedback-in #1(w152) -> ()
        n84 = Subtract(x=w152, y=w153) -> (x-y=→"ms to process":u32)
        n85 = Array To Cluster(array=w133) -> (cluster=w132:T33)
        n86 = Unbundle By Name(w132) -> ("Sorted Scores[0]"=w131:T34)
        n87 = Unbundle By Name(w128) -> ("Normalized Rect"=w127:T35)
        n88 = Unbundle By Name(w127) -> ("Numeric 2"=→"RightSide":dbl, "Numeric 5"=→"LeftSide":dbl)  [unwired: 1 out]
        n89 = Unbundle By Name(w131) -> ("Scale"=→"Scale":dbl)
        "Mbps" <- w162
        "fps" <- w161
        "Template 2" <- w134
      }
    }
  }
  n90 = register-events(refnum<vi> refnum) -> (reference out=w52:refnum<event-registration>, error out=w51:errorcluster)  [unwired: 2 in]
  n91 = property class="VI"() -> ("Panel"=w55:refnum<vi>)  [unwired: 2 in, 2 out]
  n92 = while {
    tunnel: w44 -> [w206]
    tunnel: w23 -> [w204]
    tunnel: [w202] -> _
    tunnel: u32 1000 ("milliseconds to wait") -> [w201]
    i -> [w202]
    stop <- FALSE stop-if-true
    n93 = local read "Rec Mode"() -> (w197:enum32{"Stop", "Record", "Playback"})
    n94 = Wait on Notification(notifier=w204, timeout in ms (-1)=w201) -> (notification=w203:string, timed out?=w199:bool)  [unwired: 2 in, 2 out]
    n95 = Equal?(x=w197, y=u16 2 ("Rec Mode")) -> (x = y?=w198:bool)
    n96 = Compound Arithmetic op=OR(invert w199, w198) -> (w200:bool)
    n97 = case shown="True" w200 {
      tunnel: w206 -> [_ w209]
      tunnel: w203 -> [_ w208]
      tunnel: "Dashboard" -> [_ w207]
      frame False {
      }
      frame True {
        n98 = call <vilib>:"Bind Controls to SmartDashboard.vi"("Client Name"=w207, "Bound Control Refs"=w209, "Server IP Address"=w208) -> ()  [unwired: 9 in]
      }
    }
  }
  n99 = vi-ref "Playback Controls.vi"() -> (w53:refnum<vi>)
  n100 = call "Initialize Camera and CheckList.vi"("ListBox in"=w35) -> ("Cluster"=w59:cluster{"value":i32, "value":i32, "index":i32}, "Array"=w60:cluster{string[]}[], "File Refnum"=w58:T36)  [unwired: 8 in]
  n101 = property class="Pnl"(reference=w55) -> ("Panes[]"=w56:refnum<vi>[])  [unwired: 1 in, 2 out]
  n102 = property on="Camera Settings" class="Clust (strict)"("Val(Sgnl)"=w59) -> ()  [unwired: 2 in, 2 out]
  n103 = Index Array(array=w56) -> (element=w54:refnum<vi>)  [unwired: 1 in]
  n104 = control-ref of="Test Tree"() -> (w57:refnum<vi>)
  n105 = while {
    tunnel: w60 -> [w217]
    shift-right: [w216] -> _
    shift-left: w58 -> [w215]
    tunnel: [w214] -> _
    tunnel: w57 -> [w213]
    tunnel: w53 -> [w212]
    tunnel: w52 -> [w211]
    tunnel: w51 -> [_]
    tunnel: w47 -> [w210]
    i -> [w214]
    stop <- FALSE stop-if-true
    n106 = event shown="[0] Timeout" {
      selector: w211 -> [_ _ _ _ _ _ _ _ _ _ _ _ _ _ _ _ _]
      dyn-events: [_ _ _ _ _ _ _ _ _ _ _ _ _ w455 _ _ _] -> _
      timeout: u32 60 ("milliseconds to wait") -> [_ _ _ _ _ _ _ _ _ _ _ _ _ _ _ _ _]
      tunnel: w213 -> [w229 _ _ _ _ _ _ _ _ _ _ _ _ _ _ _ _]
      tunnel: "Test Tree" -> [_ _ _ _ _ _ _ _ w424 w432 w434 w438 w446 _ _ _ _]
      tunnel: w217 -> [_ w251 _ _ _ _ w388 w418 _ _ _ _ _ _ _ _ _]
      tunnel: [w225 w250 w349 w354 w362 w374 w387 w411 w423 w430 w433 w437 w445 w457 w471 w472 w482] -> w216
      tunnel: w215 -> [w225 w250 w349 w354 w362 w374 w386 w411 w423 w430 w433 w437 w445 w457 w471 w472 w482]
      tunnel: w212 -> [_ _ _ _ _ _ _ _ _ _ _ _ _ w458 _ w475 _]
      tunnel: w210 -> [_ _ _ _ _ _ _ _ _ _ _ _ _ w453 _ _ _]
      event Timeout {
        n107 = event-data() -> ()  [unwired: 1 in, 1 out]
        n108 = local read "Mode"() -> (w228:T8)
        n109 = Index Array(array=T37 [{"Operation"=enum."Clear", "Color Box"=14013909}, {"Operation"=enum."Clear", "Color Box"=14013909}, {"Operation"=enum."Clear", "Color Box"=14013909}, {"Operation"=enum."Clear", "Color Box"=14013909}, {"Operation"=enum."Update", "Color Box"=14013909}, {"Operation"=enum."Update", "Color Box"=16777215}, {"Operation"=enum."Clear", "Color Box"=14013909}, {"Operation"=enum."Clear", "Color Box"=14013909}, {"Operation"=enum."Clear", "Color Box"=14013909}], index=w228) -> (element=w223:T41)
        n110 = Unbundle(w223) -> ("Operation"=w222:enum16{"Update", "Clear"}, "Color Box"=w221:u32)
        n111 = call <vilib>:"NT Read String.vi"("Name"="TestMode/TestName") -> ("String"=w232:string)  [unwired: 9 in, 1 out]
        n112 = case shown="\"Variables\"" "Dashboard Tab" {
          tunnel: w229 -> [_ w240 _]
          tunnel: "/TestMode/Automatic/" ("Name Pattern") -> [_ w239 _]
          tunnel: w222 -> [_ w238 _]
          tunnel: [_ _ w242] -> _
          tunnel: w221 -> [_ w234 _]
          frame "Custom", Default {
          }
          frame "Test" {
            w237 = -2 ("Active Item:Row Number")
            n113 = call <vilib>:"NT Read and Format Entries as Tree.vi"("Operation"=w238, "Name Pattern"=w239, "Tree Refnum"=w240) -> ()  [unwired: 7 in, 2 out]
            n114 = property on="Test Tree" class="Tree (strict)"("Active Item Row Number"=w237, "ActiveColNum"=w237, "CellBG"=w234, "Active Item Row Number"=-1 ("Active Item:Row Number"), "CellBG"=u32 5789784 ("Color Box")) -> ()  [unwired: 2 in, 2 out]
          }
          frame "Variables" {
            n115 = control-ref of="Tree"() -> (w241:refnum<vi>)
            n116 = call <vilib>:"NT Read and Format Entries as Tree.vi"("Tree Refnum"=w241) -> ("Formatted Strings"=w242:cluster{"Name":string, "Value":string}[])  [unwired: 9 in, 1 out]
          }
        }
        n117 = case shown="Default" w232 {
          tunnel: "TestMode/TestProgress" ("Name") -> [w244 _]
          tunnel: "TestMode/TestProgressText" ("Name") -> [w243 _]
          frame Default {
            n118 = call <vilib>:"NT Read Number.vi"("Name"=w244) -> ("Numeric"=w245:dbl)  [unwired: 9 in, 1 out]
            n119 = call <vilib>:"NT Read String.vi"("Name"=w243) -> ("String"=w246:string)  [unwired: 9 in, 1 out]
            n120 = Bundle("Numeric"=w245, "String"=w246) -> (→"Progress":cluster{"Numeric":dbl, "String":string})  [unwired: 1 in]
          }
          frame "" {
            n121 = property on="Progress" class="Clust (strict)"("Visible"=FALSE) -> ()  [unwired: 2 in, 2 out]
            n122 = local write "Test Name"(u16 0) -> ()
          }
        }
      }
      event "Test Tree": Value Change {
        # "Show appropriate\ncontrols"
        n123 = event-data() -> ("CtlRef"=w254:refnum<vi>, "NewVal"=w252:string)  [unwired: 1 in]
        n124 = call <vilib>:"WPI_UtilitiesGetTreeIOName.vi"("NewVal"=w252, "TreeControl in"=w254) -> ("I/O Name"=w255:string)  [unwired: 9 in]
        n125 = case shown="\"Camera\"" w255 {
          selector: w255 -> [_ w262 _ w280 w289 _]
          tunnel: w252 -> [_ _ w277 w279 _ w296]
          tunnel: w251 -> [_ _ _ _ _ w295]
          frame Default {
            w257 = FALSE ("Visible")
            w256 = FALSE ("Visible")
            n126 = property on="Motor" class="Clust (strict)"("Visible"=w256) -> ()  [unwired: 2 in, 2 out]
            n127 = property on="Test Ring" class="Ring (strict)"("Visible"=w256) -> ()  [unwired: 2 in, 2 out]
            n128 = property on="Rev/Fwd" class="Clust (strict)"("Visible"=w257) -> ()  [unwired: 2 in, 2 out]
            n129 = property on="On/Off" class="Bool (strict)"("Visible"=w257) -> ()  [unwired: 2 in, 2 out]
            n130 = property on="Test Slider" class="Slide (strict)"("Visible"=w257) -> ()  [unwired: 2 in, 2 out]
          }
          frame "Motor", "PWM" {
            w263 = FALSE ("Visible")
            n131 = case shown="\"Motor\", Default" w262 {
              tunnel: [1.0 ("Value") -1.0 ("Value")] -> w261
              tunnel: [255.0 ("Value") 1.0 ("Value")] -> w260
              tunnel: [128.0 ("Value") 0.0 ("Value")] -> w259
              tunnel: [64.0 ("Value") 0.5 ("Value")] -> w258
              frame "PWM" {
              }
              frame "Motor", Default {
              }
            }
            n132 = property on="Motor" class="Clust (strict)"("Visible"=TRUE) -> ()  [unwired: 2 in, 2 out]
            n133 = property on="Value" class="Slide (strict)"("Value"=w259, "Scale.Minimum"=w261, "Scale.Maximum"=w260, "Scale.Increment"=w258) -> ()  [unwired: 2 in, 2 out]
            n134 = property on="On/Off" class="Bool (strict)"("Visible"=w263) -> ()  [unwired: 2 in, 2 out]
            n135 = property on="Test Slider" class="Slide (strict)"("Visible"=w263) -> ()  [unwired: 2 in, 2 out]
            n136 = property on="Test Ring" class="Ring (strict)"("Visible"=w263) -> ()  [unwired: 2 in, 2 out]
            n137 = property on="Rev/Fwd" class="Clust (strict)"("Visible"=w263) -> ()  [unwired: 2 in, 2 out]
          }
          frame "Servo" {
            w275 = FALSE ("Visible")
            n138 = call <vilib>:"NT Read Number.vi"("Name"=w277) -> ("Numeric"=w276:dbl)  [unwired: 9 in, 1 out]
            n139 = property on="Test Slider" class="Slide (strict)"("Visible"=TRUE, "Scale.Maximum"=170.0 ("Scale.Range:Maximum")) -> ()  [unwired: 2 in, 2 out]
            n140 = local write "Test Slider"(w276) -> ()
            n141 = property on="Motor" class="Clust (strict)"("Visible"=w275) -> ()  [unwired: 2 in, 2 out]
            n142 = property on="Rev/Fwd" class="Clust (strict)"("Visible"=w275) -> ()  [unwired: 2 in, 2 out]
            n143 = property on="On/Off" class="Bool (strict)"("Visible"=w275) -> ()  [unwired: 2 in, 2 out]
            n144 = property on="Test Ring" class="Ring (strict)"("Visible"=w275) -> ()  [unwired: 2 in, 2 out]
          }
          frame "Relay", "Solenoid" {
            w278 = FALSE ("Visible")
            n145 = property on="Motor" class="Clust (strict)"("Visible"=w278) -> ()  [unwired: 2 in, 2 out]
            n146 = property on="Test Slider" class="Slide (strict)"("Visible"=w278) -> ()  [unwired: 2 in, 2 out]
            n147 = Search and Replace String(input string=w279, search string="/Value  **", replace string="/Direction") -> (result string=w285:string)  [unwired: 5 in, 3 out]
            n148 = property on="Test Ring" class="Ring (strict)"("Visible"=w278) -> ()  [unwired: 2 in, 2 out]
            n149 = call <vilib>:"NT Read String.vi"("Name"=w285) -> ("String"=w283:string)  [unwired: 9 in, 1 out]
            n150 = Equal?(x="Both directions", y=w283) -> (x = y?=w281:bool)
            n151 = Not(x=w281) -> (.not. x?=w282:bool)
            n152 = property on="Rev/Fwd" class="Clust (strict)"("Visible"=w281) -> ()  [unwired: 2 in, 2 out]
            n153 = property on="On/Off" class="Bool (strict)"("Visible"=w282, "Caption.Text"=w280) -> ()  [unwired: 2 in, 2 out]
          }
          frame "Compressor", "Digital Out" {
            w288 = FALSE ("Visible")
            # "Get direction and finish"
            n154 = property on="Motor" class="Clust (strict)"("Visible"=w288) -> ()  [unwired: 2 in, 2 out]
            n155 = property on="Test Slider" class="Slide (strict)"("Visible"=w288) -> ()  [unwired: 2 in, 2 out]
            n156 = property on="Test Ring" class="Ring (strict)"("Visible"=w288) -> ()  [unwired: 2 in, 2 out]
            n157 = property on="On/Off" class="Bool (strict)"("Visible"=TRUE, "Caption.Text"=w289) -> ()  [unwired: 2 in, 2 out]
            n158 = property on="Rev/Fwd" class="Clust (strict)"("Visible"=FALSE) -> ()  [unwired: 2 in, 2 out]
          }
          frame "Camera" {
            n159 = call <vilib>:"Get Last Path Segment.vi"("String in"=w296) -> ("String out"=w297:string)  [unwired: 10 in]
            n160 = property on="On/Off" class="Bool (strict)"("Visible"=FALSE) -> ()  [unwired: 2 in, 2 out]
            n161 = property on="Motor" class="Clust (strict)"("Visible"=FALSE) -> ()  [unwired: 2 in, 2 out]
            n162 = property on="Rev/Fwd" class="Clust (strict)"("Visible"=FALSE) -> ()  [unwired: 2 in, 2 out]
            n163 = case shown="\"White Balance  **\"" w297 {
              tunnel: w296 -> [w303 w312 w321 w330 w339 _ w345]
              tunnel: w295 -> [w301 w309 w318 w327 w336 _ _]
              frame "Size  **" {
                n164 = Index Array(array=w301) -> (element=w300:cluster{string[]})  [unwired: 1 in]
                n165 = call <vilib>:"NT Read String.vi"("Name"=w303) -> ("String"=w302:string)  [unwired: 9 in, 1 out]
                n166 = Unbundle(w300) -> (w298:string[])
                n167 = Match First String(2:w298, 3:w302) -> (0:w299:i32)  [unwired: 1 out]
                n168 = property on="Test Ring" class="Ring (strict)"("Value"=w299, "Strings []"=w298) -> ()  [unwired: 2 in, 2 out]
                n169 = property on="Test Ring" class="Ring (strict)"("Visible"=TRUE) -> ()  [unwired: 2 in, 2 out]
                n170 = property on="Test Slider" class="Slide (strict)"("Visible"=FALSE) -> ()  [unwired: 2 in, 2 out]
              }
              frame "White Balance  **" {
                n171 = Index Array(array=w309, index=1) -> (element=w310:cluster{string[]})
                n172 = call <vilib>:"NT Read String.vi"("Name"=w312) -> ("String"=w311:string)  [unwired: 9 in, 1 out]
                n173 = Unbundle(w310) -> (w307:string[])
                n174 = Match First String(2:w307, 3:w311) -> (0:w306:i32)  [unwired: 1 out]
                n175 = property on="Test Ring" class="Ring (strict)"("Value"=w306, "Strings []"=w307) -> ()  [unwired: 2 in, 2 out]
                n176 = property on="Test Ring" class="Ring (strict)"("Visible"=TRUE) -> ()  [unwired: 2 in, 2 out]
                n177 = property on="Test Slider" class="Slide (strict)"("Visible"=FALSE) -> ()  [unwired: 2 in, 2 out]
              }
              frame "Exposure  **" {
                n178 = Index Array(array=w318, index=2) -> (element=w319:cluster{string[]})
                n179 = call <vilib>:"NT Read String.vi"("Name"=w321) -> ("String"=w320:string)  [unwired: 9 in, 1 out]
                n180 = Unbundle(w319) -> (w315:string[])
                n181 = Match First String(2:w315, 3:w320) -> (0:w316:i32)  [unwired: 1 out]
                n182 = property on="Test Ring" class="Ring (strict)"("Value"=w316, "Strings []"=w315) -> ()  [unwired: 2 in, 2 out]
                n183 = property on="Test Ring" class="Ring (strict)"("Visible"=TRUE) -> ()  [unwired: 2 in, 2 out]
                n184 = property on="Test Slider" class="Slide (strict)"("Visible"=FALSE) -> ()  [unwired: 2 in, 2 out]
              }
              frame "Exposure Priority  **" {
                n185 = Index Array(array=w327, index=3) -> (element=w328:cluster{string[]})
                n186 = call <vilib>:"NT Read String.vi"("Name"=w330) -> ("String"=w329:string)  [unwired: 9 in, 1 out]
                n187 = Unbundle(w328) -> (w324:string[])
                n188 = Match First String(2:w324, 3:w329) -> (0:w325:i32)  [unwired: 1 out]
                n189 = property on="Test Ring" class="Ring (strict)"("Value"=w325, "Strings []"=w324) -> ()  [unwired: 2 in, 2 out]
                n190 = property on="Test Ring" class="Ring (strict)"("Visible"=TRUE) -> ()  [unwired: 2 in, 2 out]
                n191 = property on="Test Slider" class="Slide (strict)"("Visible"=FALSE) -> ()  [unwired: 2 in, 2 out]
              }
              frame "Color Enable  **" {
                n192 = Index Array(array=w336, index=4) -> (element=w337:cluster{string[]})
                n193 = call <vilib>:"NT Read String.vi"("Name"=w339) -> ("String"=w338:string)  [unwired: 9 in, 1 out]
                n194 = Unbundle(w337) -> (w333:string[])
                n195 = Match First String(2:w333, 3:w338) -> (0:w334:i32)  [unwired: 1 out]
                n196 = property on="Test Ring" class="Ring (strict)"("Value"=w334, "Strings []"=w333) -> ()  [unwired: 2 in, 2 out]
                n197 = property on="Test Ring" class="Ring (strict)"("Visible"=TRUE) -> ()  [unwired: 2 in, 2 out]
                n198 = property on="Test Slider" class="Slide (strict)"("Visible"=FALSE) -> ()  [unwired: 2 in, 2 out]
              }
              frame Default {
                n199 = property on="Test Ring" class="Ring (strict)"("Visible"=FALSE) -> ()  [unwired: 2 in, 2 out]
                n200 = property on="Test Slider" class="Slide (strict)"("Visible"=FALSE) -> ()  [unwired: 2 in, 2 out]
              }
              frame "Brightness  **", "Color Level  **", "Compression  **", "FPS  **", "Sharpness  **" {
                n201 = call <vilib>:"NT Read Number.vi"("Name"=w345) -> ("Numeric"=w344:dbl)  [unwired: 9 in, 1 out]
                n202 = local write "Test Slider"(w344) -> ()
                n203 = property on="Test Slider" class="Slide (strict)"("Visible"=TRUE, "Scale.Maximum"=100.0 ("Scale.Range:Maximum")) -> ()  [unwired: 2 in, 2 out]
                n204 = property on="Test Ring" class="Ring (strict)"("Visible"=FALSE) -> ()  [unwired: 2 in, 2 out]
              }
            }
          }
        }
        n205 = property on="Progress" class="Clust (strict)"("Visible"=FALSE) -> ()  [unwired: 2 in, 2 out]
      }
      event "Test Name": Mouse Enter {
        # "Populate the ring with the list of tests"
        n206 = event-data() -> ()  [unwired: 1 in, 1 out]
        n207 = call <vilib>:"NT Read String Array.vi"("Name"="TestMode/TestList") -> ("String Array"=w353:string[])  [unwired: 9 in, 1 out]
        n208 = Build Array (concatenate)("Select the test to run...", w353) -> (w352:string[])
        n209 = property on="Test Name" class="Ring (strict)"("Strings []"=w352) -> ()  [unwired: 2 in, 2 out]
      }
      event "Test Name": Value Change {
        w355 = FALSE ("Visible")
        # "Tell the robot the test name to run"
        n210 = event-data() -> ("NewVal"=w359:u16)  [unwired: 1 in]
        n211 = property on="Test Name" class="Ring (strict)"() -> ("Strings []"=w360:string[])  [unwired: 2 in, 2 out]
        n212 = local write "Progress"(T12 {"Test Progress"=0, "Test Progress Text"=""} ("Progress")) -> ()
        n213 = Index Array(array=w360, index=w359) -> (element=w358:string)
        n214 = call <vilib>:"NT Write String.vi"("String"=w358, "Name"="TestMode/TestName") -> ()  [unwired: 9 in, 1 out]
        n215 = property on="Progress" class="Clust (strict)"("Visible"=TRUE) -> ()  [unwired: 2 in, 2 out]
        n216 = property on="Motor" class="Clust (strict)"("Visible"=w355) -> ()  [unwired: 2 in, 2 out]
        n217 = property on="Test Slider" class="Slide (strict)"("Visible"=w355) -> ()  [unwired: 2 in, 2 out]
        n218 = property on="On/Off" class="Bool (strict)"("Visible"=w355) -> ()  [unwired: 2 in, 2 out]
        n219 = property on="Rev/Fwd" class="Clust (strict)"("Visible"=w355) -> ()  [unwired: 2 in, 2 out]
        n220 = property on="Test Ring" class="Ring (strict)"("Visible"=w355) -> ()  [unwired: 2 in, 2 out]
      }
      event "Listbox": Double Click {
        # "Shift clears all"
        # "Update symbols on the listbox"
        n221 = event-data() -> ("PlatMods.Shift"=w363:bool, "Row"=w365:i32)  [unwired: 1 in]
        n222 = case shown="True" w363 {
          tunnel: w365 -> [w369 _]
          tunnel: 1 -> [w368 _]
          frame False {
            n223 = property on="Listbox" class="LstBox (strict)"() -> ("Item Symbols"=w367:i32[])  [unwired: 2 in, 2 out]
            n224 = Replace Array Subset(array=w367, new element=w368, index=w369) -> (w366:i32[])
            n225 = property on="Listbox" class="LstBox (strict)"("Item Symbols"=w366) -> ()  [unwired: 2 in, 2 out]
          }
          frame True {
            w370 = 0 ("Top Row")
            n226 = property on="Listbox" class="LstBox (strict)"() -> ("Number of Rows"=w372:u32)  [unwired: 2 in, 2 out]
            n227 = Initialize Array(0, w372) -> (w371:i32[])
            n228 = property on="Listbox" class="LstBox (strict)"("Top Row"=w370, "Value"=w370, "Item Symbols"=w371) -> ()  [unwired: 2 in, 2 out]
          }
        }
      }
      event "Listbox": Key Down {
        # "Update symbols on the listbox\nLeft and right keys check and uncheck"
        n229 = event-data() -> ("VKey"=w376:T38)  [unwired: 1 in]
        n230 = case shown="\"Left\", \"Right\"" w376 {
          selector: w376 -> [w381 _]
          tunnel: eventvkey."Left" ("VKey") -> [w379 _]
          frame "Left", "Right" {
            n231 = Equal?(x=w379, y=w381) -> (x = y?=w380:bool)
            n232 = Select(t=0, s=w380, f=1) -> (s? t:f=w382:i32)
            n233 = property on="Listbox" class="LstBox (strict)"() -> ("Item Symbols"=w385:i32[])  [unwired: 2 in, 2 out]
            n234 = Replace Array Subset(array=w385, new element=w382, index="Listbox") -> (w384:i32[])
            n235 = property on="Listbox" class="LstBox (strict)"("Item Symbols"=w384) -> ()  [unwired: 2 in, 2 out]
          }
          frame Default {
          }
        }
      }
      event "DB Camera Config": Value Change {
        # "Show or hide the cluster of controls, store in ini file"
        n236 = event-data() -> ("NewVal"=w389:bool)  [unwired: 1 in]
        n237 = case shown="False" w389 {
          tunnel: w388 -> [w398 _]
          tunnel: [w391 w409] -> w387
          tunnel: w386 -> [w390 w409]
          frame False {
            w405 = "Camera"
            w408 = FALSE ("Visible")
            n238 = local read "Camera Settings"() -> (w397:T4)
            n239 = Index Array(array=w398) -> (element=w401:cluster{string[]})  [unwired: 1 in]
            n240 = Unbundle(w397) -> ("Frame Rate"=w396:i32, "Compression"=w395:i32, "Size"=w399:u16)
            n241 = Unbundle(w401) -> (w400:string[])
            n242 = Index Array(array=w400, index=w399) -> (element=w394:string)
            n243 = call-poly <vilib>:"Write Key.vi"("section"=w405, "value"=w394, "key"="Size", "refnum"=w390) -> ("refnum out"=w407:T36)  [unwired: 2 in, 5 out]
            n244 = call-poly <vilib>:"Write Key.vi"("section"=w405, "value"=w396, "key"="FrameRate", "refnum"=w407) -> ("refnum out"=w406:T36)  [unwired: 1 in, 6 out]
            n245 = property on="Camera Settings" class="Clust (strict)"("Visible"=w408) -> ()  [unwired: 2 in, 2 out]
            n246 = local write "DB Camera Config"(w408) -> ()
            n247 = call-poly <vilib>:"Write Key.vi"("section"=w405, "value"=w395, "key"="Compression", "refnum"=w406) -> ("refnum out"=w392:T36)  [unwired: 1 in, 6 out]
            n248 = call <vilib>:"Close Config Data.vi"("refnum"=w392) -> ("file path"=w393:path)  [unwired: 2 in, 8 out]
            n249 = call <vilib>:"Open Config Data.vi"("configuration file path"=w393) -> ("refnum"=w391:T36)  [unwired: 8 in, 2 out]
          }
          frame True {
            n250 = property on="Camera Settings" class="Clust (strict)"("Visible"=TRUE) -> ()  [unwired: 2 in, 2 out]
          }
        }
      }
      event "Camera Settings": Value Change {
        # "Update summary string when any elements of DB camera change"
        n251 = event-data() -> ("NewVal"=w422:T4)  [unwired: 1 in]
        n252 = Index Array(array=w418) -> (element=w417:cluster{string[]})  [unwired: 1 in]
        n253 = Unbundle(w422) -> ("Frame Rate"=w413:i32, "Compression"=w412:i32, "Size"=w415:u16)
        n254 = Unbundle(w417) -> (w416:string[])
        n255 = Index Array(array=w416, index=w415) -> (element=w414:string)
        n256 = Format Into String(format string="%s   %dfps   %d%%", w414, w413, w412) -> (resulting string=w419:string)  [unwired: 2 in, 1 out]
        n257 = Build Array(w419) -> (w420:string[])
        n258 = property on="DB Camera Config" class="Bool (strict)"("Strings [4]"=w420) -> ()  [unwired: 2 in, 2 out]
      }
      event "Motor.Enable": Value Change {
        # "When the test mode otor enable helper is set, update that\ntree row item's value"
        n259 = event-data() -> ("NewVal"=w428:bool)  [unwired: 1 in]
        n260 = Unbundle("Motor") -> ("Value"=w427:dbl)  [unwired: 1 out]
        n261 = Select(t=w427, s=w428, f=0.0) -> (s? t:f=w425:dbl)
        n262 = call <vilib>:"NT Write Number.vi"("Numeric"=w425, "Name"=w424) -> ()  [unwired: 9 in, 1 out]
      }
      event "Test Slider": Value Change {
        # "When the test mode slider helper is set, update that\ntree row item's value"
        n263 = event-data() -> ("NewVal"=w431:dbl)  [unwired: 1 in]
        n264 = call <vilib>:"NT Write Number.vi"("Numeric"=w431, "Name"=w432) -> ()  [unwired: 9 in, 1 out]
      }
      event "On/Off": Value Change {
        # "When the test mode on/off helper value is set, update that\ntree row item's value"
        n265 = event-data() -> ("NewVal"=w436:bool)  [unwired: 1 in]
        n266 = Boolean To (0,1)(Boolean=w436) -> (0, 1=w435:i16)
        n267 = call <vilib>:"NT Write Number.vi"("Numeric"=w435, "Name"=w434) -> ()  [unwired: 9 in, 1 out]
      }
      event "Rev/Fwd": Value Change {
        # "When the test mode helper value for relays is set, update that\ntree row item's value"
        n268 = event-data() -> ("NewVal.Forward"=w444:bool, "NewVal.Reverse"=w443:bool)  [unwired: 1 in]
        n269 = Boolean To (0,1)(Boolean=w444) -> (0, 1=w440:i16)
        n270 = Boolean To (0,1)(Boolean=w443) -> (0, 1=w442:i16)
        n271 = Negate(x=w442) -> (-x=w441:i16)
        n272 = Add(x=w440, y=w441) -> (x+y=w439:i16)
        n273 = call <vilib>:"NT Write Number.vi"("Numeric"=w439, "Name"=w438) -> ()  [unwired: 9 in, 1 out]
      }
      event "Test Ring": Value Change {
        # "When a test mode helper value is selected from the ring,\nset the tree item's variable to the string value"
        n274 = event-data() -> ("NewVal"=w448:u16)  [unwired: 1 in]
        n275 = property on="Test Ring" class="Ring (strict)"() -> ("Strings []"=w449:string[])  [unwired: 2 in, 2 out]
        n276 = Index Array(array=w449, index=w448) -> (element=w447:string)
        n277 = call <vilib>:"NT Write String.vi"("String"=w447, "Name"=w446) -> ()  [unwired: 9 in, 1 out]
      }
      event "Rec Mode": Value Change {
        # "Update globals for recording mode and path to read log from.\nClear when logging and let NetworkTables set path for vision to\nuse."
        n278 = event-data() -> ("NewVal"=w459:enum32{"Stop", "Record", "Playback"})  [unwired: 1 in]
        n279 = global write "WPI_DashboardLogging Global.vi" "Logging Filename"(path "") -> ()
        n280 = case shown="\"Playback\"" w459 {
          tunnel: w458 -> [_ w461 w469]
          tunnel: [_ _ w468] -> w455
          tunnel: [_ _ w467] -> _
          tunnel: w453 -> [_ _ w465]
          tunnel: cluster{i32, i32} {-250, 170} -> [_ _ w464]
          tunnel: [_ _ T39 {"Image Size"=TRUE, "Image Type"=TRUE, "Pixel Value"=TRUE, "ROI Information"=TRUE, "Zoom Factor"=FALSE} ("Image Information Shown:All Elements")] -> w451
          tunnel: [_ _ TRUE ("Zoom Factor")] -> w450
          frame Default {
          }
          frame "Stop", "Record" {
            # "Place Window too"
            n281 = invoke class="VI" method="FP.Close"(reference=w461) -> (reference out=w460:refnum<vi>)  [unwired: 2 in, 2 out]
            n282 = invoke class="VI" method="Abort VI"(reference=w460) -> ()  [unwired: 2 in, 3 out]
          }
          frame "Playback" {
            n283 = call "Open Playback Panel.vi"("Offset"=w464, "DB VI Ref"=w465, "Playback in"=w469) -> ("Playback out"=w466:refnum<vi>)  [unwired: 8 in]
            n284 = register-events(w466) -> (reference out=w468:refnum<event-registration>, error out=w467:errorcluster)  [unwired: 2 in]
          }
        }
        n285 = global write "WPI_DashboardLogging Global.vi" "Recording"(w459) -> ()
        n286 = property on="Camera Image" class="ImageControl"("Image Information Shown"=w451, "Image Information Visible"=w450) -> ()  [unwired: 2 in, 2 out]
        n287 = call <vilib>:"WPI_DashboardNT Log FieldName Cache.vi"("Operation"=enum16{"Lookup/Add", "Index", "Clear"}."Clear") -> ()  [unwired: 8 in, 3 out]
      }
      event Panel Close {
        w470 = enum32{"Stop", "Record", "Playback"}."Stop" ("Rec Mode")
        # "Playback window has been closed, abort"
        n288 = event-data() -> ()  [unwired: 1 in, 4 out]
        n289 = local write "Rec Mode"(w470) -> ()
        n290 = global write "WPI_DashboardLogging Global.vi" "Recording"(w470) -> ()
      }
      event Panel Close {
        # "Abort playback window and ourself"
        n291 = event-data() -> ()  [unwired: 1 in, 4 out]
        n292 = invoke class="VI" method="FP.Close"(reference=w475) -> (reference out=w474:refnum<vi>)  [unwired: 2 in, 2 out]
        n293 = invoke class="VI" method="Abort VI"(reference=w474) -> (error out=w473:errorcluster)  [unwired: 2 in, 2 out]
        n294 = invoke class="VI" method="Abort VI"(error in=w473) -> ()  [unwired: 2 in, 3 out]
      }
      event "Vision": Value Change {
        # "Enable/Disable Compression slider.\nHW USB is hard-coded into the camera"
        n295 = event-data() -> ("NewVal"=w481:u16)  [unwired: 1 in]
        n296 = Equal?(x=w481, y=u32 2 ("milliseconds to wait")) -> (x = y?=w479:bool)
        n297 = Select(t=T40."Disabled and Grayed Out" ("Disabled"), s=w479, f=T40."Enabled" ("Disabled")) -> (s? t:f=w476:T40)
        n298 = property on="Compression" class="Slide (strict)"("DisabledEnum"=w476) -> ()  [unwired: 2 in, 2 out]
      }
    }
  }
  n299 = while {
    tunnel: w54 -> [w484]
    i -> [w487]
    stop <- FALSE stop-if-true
    n300 = Wait (ms)(milliseconds to wait=u32 100) -> ()  [unwired: 1 out]
    n301 = case shown="\"Playback\"" "Rec Mode" {
      tunnel: w487 -> [_ _ w502]
      tunnel: [u32 2829099 ("Base Color") u32 11141120 ("Target Color") w491] -> w483
      frame "Stop", Default {
        # "Reset the color, extra updates don't cost much"
      }
      frame "Record" {
      }
      frame "Playback" {
        # "Playback"
        n302 = Quotient & Remainder(x=w502, y=u32 50 ("milliseconds to wait")) -> (x-y*floor(x/y)=w498:u32)  [unwired: 1 out]
        n303 = Divide(x=w498, y=u32 50 ("milliseconds to wait")) -> (x/y=w495:dbl)
        n304 = Multiply(x=6.283185307179586, y=w495) -> (x*y=w500:dbl)
        n305 = Sine(x=w500) -> (sin(x)=w499:dbl)
        n306 = Absolute Value(x=w499) -> (abs(x)=w492:dbl)
        n307 = call "Interpolate RGB Color.vi"("Proportion"=w492, "Target Color"=u32 30976, "Base Color"=u32 2829099) -> ("Result Color"=w491:u32)  [unwired: 8 in]
      }
    }
    n308 = property class="Pane"(reference=w484, "PaneColor"=w483) -> ()  [unwired: 1 in, 2 out]
  }
  n309 = TCP Create Listener(10:u16 1741 ("timeout ms (25000)")) -> (3:w19:refnum<k5>)  [unwired: 4 in, 2 out]
  n310 = while {
    tunnel: w19 -> [w504]
    stop <- FALSE stop-if-true
    n311 = TCP Wait On Listener(11:w504) -> (4:w503:refnum<k5>)  [unwired: 3 in, 4 out]
    n312 = local write "TCP"(w503) -> ()
  }
  n313 = property on="On/Off" class="Bool (strict)"("Visible"=w24) -> ()  [unwired: 2 in, 2 out]
  n314 = property on="Motor" class="Clust (strict)"("Visible"=w24) -> ()  [unwired: 2 in, 2 out]
  n315 = property on="Progress" class="Clust (strict)"("Visible"=w24) -> ()  [unwired: 2 in, 2 out]
  n316 = property on="Test Ring" class="Ring (strict)"("Visible"=w24) -> ()  [unwired: 2 in, 2 out]
  n317 = property on="Rev/Fwd" class="Clust (strict)"("Visible"=w24) -> ()  [unwired: 2 in, 2 out]
  n318 = property on="Camera Settings" class="Clust (strict)"("Visible"=w24) -> ()  [unwired: 2 in, 2 out]
  n319 = local write "DB Camera Config"(w24) -> ()
  n320 = global write "WPI_DashboardLogging Global.vi" "Recording"(w48) -> ()
  n321 = local write "Rec Mode"(w48) -> ()
